vi "App - analyze RUS V6.vi"() -> ()   [LabVIEW 2018] (continued)
5_Cooling_2nd_try/September_2014/091614/102.64400K_500_2500_2.10000V_0.00000T_Sep16-2014__21-41-37_001_091614.bin", "last mod"=timestamp(3493762897 s since 1904-01-01), "file name str"="D:\\Data\\Ultrasound\\LSCO\\LSCO22__130814c\\5_Cooling_2nd_try\\September_2014\\091614\\102.64400K_500_2500_2.10000V_0.00000T_Sep16-2014__21-41-37_001_091614.bin", "mod time(min)"=58229381.61666667, "file format"=enum."binary", "power(V)"=2.1, "Magn Field(T) "=0.0}, {"temperature"=102.47, "temperature str"="102.47000", "file path"=path "D:/Data/Ultrasound/LSCO/LSCO22__130814c/5_Cooling_2nd_try/September_2014/091614/102.47000K_500_2500_2.10000V_0.00000T_Sep16-2014__21-42-56_001_091614.bin", "last mod"=timestamp(3493762976 s since 1904-01-01), "file name str"="D:\\Data\\Ultrasound\\LSCO\\LSCO22__130814c\\5_Cooling_2nd_try\\September_2014\\091614\\102.47000K_500_2500_2.10000V_0.00000T_Sep16-2014__21-42-56_001_091614.bin", "mod time(min)"=58229382.93333333, "file format"=enum."binary", "power(V)"=2.1, "Magn Field(T) "=0.0}, {"temperature"=102.285, "temperature str"="102.28500", "file path"=path "D:/Data/Ultrasound/LSCO/LSCO22__130814c/5_Cooling_2nd_try/September_2014/091614/102.28500K_500_2500_2.10000V_0.00000T_Sep16-2014__21-44-15_001_091614.bin", "last mod"=timestamp(3493763055 s since 1904-01-01), "file name str"="D:\\Data\\Ultrasound\\LSCO\\LSCO22__130814c\\5_Cooling_2nd_try\\September_2014\\091614\\102.28500K_500_2500_2.10000V_0.00000T_Sep16-2014__21-44-15_001_091614.bin", "mod time(min)"=58229384.25, "file format"=enum."binary", "power(V)"=2.1, "Magn Field(T) "=0.0}, {"temperature"=102.107, "temperature str"="102.10700", "file path"=path "D:/Data/Ultrasound/LSCO/LSCO22__130814c/5_Cooling_2nd_try/September_2014/091614/102.10700K_500_2500_2.10000V_0.00000T_Sep16-2014__21-45-35_001_091614.bin", "last mod"=timestamp(3493763135 s since 1904-01-01), "file name str"="D:\\Data\\Ultrasound\\LSCO\\LSCO22__130814c\\5_Cooling_2nd_try\\September_2014\\091614\\102.10700K_500_2500_2.10000V_0.00000T_Sep16-2014__21-45-35_001_091614.bin", "mod time(min)"=58229385.583333336, "file format"=enum."binary", "power(V)"=2.1, "Magn Field(T) "=0.0}, {"temperature"=101.933, "temperature str"="101.93300", "file path"=path "D:/Data/Ultrasound/LSCO/LSCO22__130814c/5_Cooling_2nd_try/September_2014/091614/101.93300K_500_2500_2.10000V_0.00000T_Sep16-2014__21-46-54_001_091614.bin", "last mod"=timestamp(3493763214 s since 1904-01-01), "file name str"="D:\\Data\\Ultrasound\\LSCO\\LSCO22__130814c\\5_Cooling_2nd_try\\September_2014\\091614\\101.93300K_500_2500_2.10000V_0.00000T_Sep16-2014__21-46-54_001_091614.bin", "mod time(min)"=58229386.9, "file format"=enum."binary", "power(V)"=2.1, "Magn Field(T) "=0.0}, {"temperature"=101.753, "temperature str"="101.75300", "file path"=path "D:/Data/Ultrasound/LSCO/LSCO22__130814c/5_Cooling_2nd_try/September_2014/091614/101.75300K_500_2500_2.10000V_0.00000T_Sep16-2014__21-48-14_001_091614.bin", "last mod"=timestamp(3493763294 s since 1904-01-01), "file name str"="D:\\Data\\Ultrasound\\LSCO\\LSCO22__130814c\\5_Cooling_2nd_try\\September_2014\\091614\\101.75300K_500_2500_2.10000V_0.00000T_Sep16-2014__21-48-14_001_091614.bin", "mod time(min)"=58229388.233333334, "file format"=enum."binary", "power(V)"=2.1, "Magn Field(T) "=0.0}, {"temperature"=101.581, "temperature str"="101.58100", "file path"=path "D:/Data/Ultrasound/LSCO/LSCO22__130814c/5_Cooling_2nd_try/September_2014/091614/101.58100K_500_2500_2.10000V_0.00000T_Sep16-2014__21-49-33_001_091614.bin", "last mod"=timestamp(3493763373 s since 1904-01-01), "file name str"="D:\\Data\\Ultrasound\\LSCO\\LSCO22__130814c\\5_Cooling_2nd_try\\September_2014\\091614\\101.58100K_500_2500_2.10000V_0.00000T_Sep16-2014__21-49-33_001_091614.bin", "mod time(min)"=58229389.55, "file format"=enum."binary", "power(V)"=2.1, "Magn Field(T) "=0.0}, {"temperature"=101.405, "temperature str"="101.40500", "file path"=path "D:/Data/Ultrasound/LSCO/LSCO22__130814c/5_Cooling_2nd_try/September_2014/091614/101.40500K_500_2500_2.10000V_0.00000T_Sep16-2014__21-50-52_001_091614.bin", "last mod"=timestamp(3493763452 s since 1904-01-01), "file name str"="D:\\Data\\Ultrasound\\LSCO\\LSCO22__130814c\\5_Cooling_2nd_try\\September_2014\\091614\\101.40500K_500_2500_2.10000V_0.00000T_Sep16-2014__21-50-52_001_091614.bin", "mod time(min)"=58229390.86666667, "file format"=enum."binary", "power(V)"=2.1, "Magn Field(T) "=0.0}, {"temperature"=101.228, "temperature str"="101.22800", "file path"=path "D:/Data/Ultrasound/LSCO/LSCO22__130814c/5_Cooling_2nd_try/September_2014/091614/101.22800K_500_2500_2.10000V_0.00000T_Sep16-2014__21-52-12_001_091614.bin", "last mod"=timestamp(3493763532 s since 1904-01-01), "file name str"="D:\\Data\\Ultrasound\\LSCO\\LSCO22__130814c\\5_Cooling_2nd_try\\September_2014\\091614\\101.22800K_500_2500_2.10000V_0.00000T_Sep16-2014__21-52-12_001_091614.bin", "mod time(min)"=58229392.2, "file format"=enum."binary", "power(V)"=2.1, "Magn Field(T) "=0.0}, {"temperature"=101.06, "temperature str"="101.06000", "file path"=path "D:/Data/Ultrasound/LSCO/LSCO22__130814c/5_Cooling_2nd_try/September_2014/091614/101.06000K_500_2500_2.10000V_0.00000T_Sep16-2014__21-53-31_001_091614.bin", "last mod"=timestamp(3493763611 s since 1904-01-01), "file name str"="D:\\Data\\Ultrasound\\LSCO\\LSCO22__130814c\\5_Cooling_2nd_try\\September_2014\\091614\\101.06000K_500_2500_2.10000V_0.00000T_Sep16-2014__21-53-31_001_091614.bin", "mod time(min)"=58229393.516666666, "file format"=enum."binary", "power(V)"=2.1, "Magn Field(T) "=0.0}, {"temperature"=100.883, "temperature str"="100.88300", "file path"=path "D:/Data/Ultrasound/LSCO/LSCO22__130814c/5_Cooling_2nd_try/September_2014/091614/100.88300K_500_2500_2.10000V_0.00000T_Sep16-2014__21-54-50_001_091614.bin", "last mod"=timestamp(3493763690 s since 1904-01-01), "file name str"="D:\\Data\\Ultrasound\\LSCO\\LSCO22__130814c\\5_Cooling_2nd_try\\September_2014\\091614\\100.88300K_500_2500_2.10000V_0.00000T_Sep16-2014__21-54-50_001_091614.bin", "mod time(min)"=58229394.833333336, "file format"=enum."binary", "power(V)"=2.1, "Magn Field(T) "=0.0}, {"temperature"=100.708, "temperature str"="100.70800", "file path"=path "D:/Data/Ultrasound/LSCO/LSCO22__130814c/5_Cooling_2nd_try/September_2014/091614/100.70800K_500_2500_2.10000V_0.00000T_Sep16-2014__21-56-10_001_091614.bin", "last mod"=timestamp(3493763770 s since 1904-01-01), "file name str"="D:\\Data\\Ultrasound\\LSCO\\LSCO22__130814c\\5_Cooling_2nd_try\\September_2014\\091614\\100.70800K_500_2500_2.10000V_0.00000T_Sep16-2014__21-56-10_001_091614.bin", "mod time(min)"=58229396.166666664, "file format"=enum."binary", "power(V)"=2.1, "Magn Field(T) "=0.0}, {"temperature"=100.542, "temperature str"="100.54200", "file path"=path "D:/Data/Ultrasound/LSCO/LSCO22__130814c/5_Cooling_2nd_try/September_2014/091614/100.54200K_500_2500_2.10000V_0.00000T_Sep16-2014__21-57-29_001_091614.bin", "last mod"=timestamp(3493763849 s since 1904-01-01), "file name str"="D:\\Data\\Ultrasound\\LSCO\\LSCO22__130814c\\5_Cooling_2nd_try\\September_2014\\091614\\100.54200K_500_2500_2.10000V_0.00000T_Sep16-2014__21-57-29_001_091614.bin", "mod time(min)"=58229397.483333334, "file format"=enum."binary", "power(V)"=2.1, "Magn Field(T) "=0.0}, {"temperature"=100.369, "temperature str"="100.36900", "file path"=path "D:/Data/Ultrasound/LSCO/LSCO22__130814c/5_Cooling_2nd_try/September_2014/091614/100.36900K_500_2500_2.10000V_0.00000T_Sep16-2014__21-58-49_001_091614.bin", "last mod"=timestamp(3493763929 s since 1904-01-01), "file name str"="D:\\Data\\Ultrasound\\LSCO\\LSCO22__130814c\\5_Cooling_2nd_try\\September_2014\\091614\\100.36900K_500_2500_2.10000V_0.00000T_Sep16-2014__21-58-49_001_091614.bin", "mod time(min)"=58229398.81666667, "file format"=enum."binary", "power(V)"=2.1, "Magn Field(T) "=0.0}, {"temperature"=100.203, "temperature str"="100.20300", "file path"=path "D:/Data/Ultrasound/LSCO/LSCO22__130814c/5_Cooling_2nd_try/September_2014/091614/100.20300K_500_2500_2.10000V_0.00000T_Sep16-2014__22-00-08_001_091614.bin", "last mod"=timestamp(3493764008 s since 1904-01-01), "file name str"="D:\\Data\\Ultrasound\\LSCO\\LSCO22__130814c\\5_Cooling_2nd_try\\September_2014\\091614\\100.20300K_500_2500_2.10000V_0.00000T_Sep16-2014__22-00-08_001_091614.bin", "mod time(min)"=58229400.13333333, "file format"=enum."binary", "power(V)"=2.1, "Magn Field(T) "=0.0}, {"temperature"=100.032, "temperature str"="100.03200", "file path"=path "D:/Data/Ultrasound/LSCO/LSCO22__130814c/5_Cooling_2nd_try/September_2014/091614/100.03200K_500_2500_2.10000V_0.00000T_Sep16-2014__22-01-27_001_091614.bin", "last mod"=timestamp(3493764087 s since 1904-01-01), "file name str"="D:\\Data\\Ultrasound\\LSCO\\LSCO22__130814c\\5_Cooling_2nd_try\\September_2014\\091614\\100.03200K_500_2500_2.10000V_0.00000T_Sep16-2014__22-01-27_001_091614.bin", "mod time(min)"=58229401.45, "file format"=enum."binary", "power(V)"=2.1, "Magn Field(T) "=0.0}, {"temperature"=99.859, "temperature str"="99.85900", "file path"=path "D:/Data/Ultrasound/LSCO/LSCO22__130814c/5_Cooling_2nd_try/September_2014/091614/99.85900K_500_2500_2.10000V_0.00000T_Sep16-2014__22-02-47_001_091614.bin", "last mod"=timestamp(3493764167 s since 1904-01-01), "file name str"="D:\\Data\\Ultrasound\\LSCO\\LSCO22__130814c\\5_Cooling_2nd_try\\September_2014\\091614\\99.85900K_500_2500_2.10000V_0.00000T_Sep16-2014__22-02-47_001_091614.bin", "mod time(min)"=58229402.78333333, "file format"=enum."binary", "power(V)"=2.1, "Magn Field(T) "=0.0}, {"temperature"=99.697, "temperature str"="99.69700", "file path"=path "D:/Data/Ultrasound/LSCO/LSCO22__130814c/5_Cooling_2nd_try/September_2014/091614/99.69700K_500_2500_2.10000V_0.00000T_Sep16-2014__22-04-06_001_091614.bin", "last mod"=timestamp(3493764246 s since 1904-01-01), "file name str"="D:\\Data\\Ultrasound\\LSCO\\LSCO22__130814c\\5_Cooling_2nd_try\\September_2014\\091614\\99.69700K_500_2500_2.10000V_0.00000T_Sep16-2014__22-04-06_001_091614.bin", "mod time(min)"=58229404.1, "file format"=enum."binary", "power(V)"=2.1, "Magn Field(T) "=0.0}, {"temperature"=99.53, "temperature str"="99.53000", "file path"=path "D:/Data/Ultrasound/LSCO/LSCO22__130814c/5_Cooling_2nd_try/September_2014/091614/99.53000K_500_2500_2.10000V_0.00000T_Sep16-2014__22-05-25_001_091614.bin", "last mod"=timestamp(3493764325 s since 1904-01-01), "file name str"="D:\\Data\\Ultrasound\\LSCO\\LSCO22__130814c\\5_Cooling_2nd_try\\September_2014\\091614\\99.53000K_500_2500_2.10000V_0.00000T_Sep16-2014__22-05-25_001_091614.bin", "mod time(min)"=58229405.416666664, "file format"=enum."binary", "power(V)"=2.1, "Magn Field(T) "=0.0}, {"temperature"=99.368, "temperature str"="99.36800", "file path"=path "D:/Data/Ultrasound/LSCO/LSCO22__130814c/5_Cooling_2nd_try/September_2014/091614/99.36800K_500_2500_2.10000V_0.00000T_Sep16-2014__22-06-45_001_091614.bin", "last mod"=timestamp(3493764405 s since 1904-01-01), "file name str"="D:\\Data\\Ultrasound\\LSCO\\LSCO22__130814c\\5_Cooling_2nd_try\\September_2014\\091614\\99.36800K_500_2500_2.10000V_0.00000T_Sep16-2014__22-06-45_001_091614.bin", "mod time(min)"=58229406.75, "file format"=enum."binary", "power(V)"=2.1, "Magn Field(T) "=0.0}, {"temperature"=99.199, "temperature str"="99.19900", "file path"=path "D:/Data/Ultrasound/LSCO/LSCO22__130814c/5_Cooling_2nd_try/September_2014/091614/99.19900K_500_2500_2.10000V_0.00000T_Sep16-2014__22-08-04_001_091614.bin", "last mod"=timestamp(3493764484 s since 1904-01-01), "file name str"="D:\\Data\\Ultrasound\\LSCO\\LSCO22__130814c\\5_Cooling_2nd_try\\September_2014\\091614\\99.19900K_500_2500_2.10000V_0.00000T_Sep16-2014__22-08-04_001_091614.bin", "mod time(min)"=58229408.06666667, "file format"=enum."binary", "power(V)"=2.1, "Magn Field(T) "=0.0}, {"temperature"=99.032, "temperature str"="99.03200", "file path"=path "D:/Data/Ultrasound/LSCO/LSCO22__130814c/5_Cooling_2nd_try/September_2014/091614/99.03200K_500_2500_2.10000V_0.00000T_Sep16-2014__22-09-24_001_091614.bin", "last mod"=timestamp(3493764564 s since 1904-01-01), "file name str"="D:\\Data\\Ultrasound\\LSCO\\LSCO22__130814c\\5_Cooling_2nd_try\\September_2014\\091614\\99.03200K_500_2500_2.10000V_0.00000T_Sep16-2014__22-09-24_001_091614.bin", "mod time(min)"=58229409.4, "file format"=enum."binary", "power(V)"=2.1, "Magn Field(T) "=0.0}, {"temperature"=98.874, "temperature str"="98.87400", "file path"=path "D:/Data/Ultrasound/LSCO/LSCO22__130814c/5_Cooling_2nd_try/September_2014/091614/98.87400K_500_2500_2.10000V_0.00000T_Sep16-2014__22-10-43_001_091614.bin", "last mod"=timestamp(3493764643 s since 1904-01-01), "file name str"="D:\\Data\\Ultrasound\\LSCO\\LSCO22__130814c\\5_Cooling_2nd_try\\September_2014\\091614\\98.87400K_500_2500_2.10000V_0.00000T_Sep16-2014__22-10-43_001_091614.bin", "mod time(min)"=58229410.71666667, "file format"=enum."binary", "power(V)"=2.1, "Magn Field(T) "=0.0}, {"temperature"=98.708, "temperature str"="98.70800", "file path"=path "D:/Data/Ultrasound/LSCO/LSCO22__130814c/5_Cooling_2nd_try/September_2014/091614/98.70800K_500_2500_2.10000V_0.00000T_Sep16-2014__22-12-02_001_091614.bin", "last mod"=timestamp(3493764722 s since 1904-01-01), "file name str"="D:\\Data\\Ultrasound\\LSCO\\LSCO22__130814c\\5_Cooling_2nd_try\\September_2014\\091614\\98.70800K_500_2500_2.10000V_0.00000T_Sep16-2014__22-12-02_001_091614.bin", "mod time(min)"=58229412.03333333, "file format"=enum."binary", "power(V)"=2.1, "Magn Field(T) "=0.0}, {"temperature"=98.551, "temperature str"="98.55100", "file path"=path "D:/Data/Ultrasound/LSCO/LSCO22__130814c/5_Cooling_2nd_try/September_2014/091614/98.55100K_500_2500_2.10000V_0.00000T_Sep16-2014__22-13-22_001_091614.bin", "last mod"=timestamp(3493764802 s since 1904-01-01), "file name str"="D:\\Data\\Ultrasound\\LSCO\\LSCO22__130814c\\5_Cooling_2nd_try\\September_2014\\091614\\98.55100K_500_2500_2.10000V_0.00000T_Sep16-2014__22-13-22_001_091614.bin", "mod time(min)"=58229413.36666667, "file format"=enum."binary", "power(V)"=2.1, "Magn Field(T) "=0.0}, {"temperature"=98.387, "temperature str"="98.38700", "file path"=path "D:/Data/Ultrasound/LSCO/LSCO22__130814c/5_Cooling_2nd_try/September_2014/091614/98.38700K_500_2500_2.10000V_0.00000T_Sep16-2014__22-14-41_001_091614.bin", "last mod"=timestamp(3493764881 s since 1904-01-01), "file name str"="D:\\Data\\Ultrasound\\LSCO\\LSCO22__130814c\\5_Cooling_2nd_try\\September_2014\\091614\\98.38700K_500_2500_2.10000V_0.00000T_Sep16-2014__22-14-41_001_091614.bin", "mod time(min)"=58229414.68333333, "file format"=enum."binary", "power(V)"=2.1, "Magn Field(T) "=0.0}, {"temperature"=98.223, "temperature str"="98.22300", "file path"=path "D:/Data/Ultrasound/LSCO/LSCO22__130814c/5_Cooling_2nd_try/September_2014/091614/98.22300K_500_2500_2.10000V_0.00000T_Sep16-2014__22-16-00_001_091614.bin", "last mod"=timestamp(3493764960 s since 1904-01-01), "file name str"="D:\\Data\\Ultrasound\\LSCO\\LSCO22__130814c\\5_Cooling_2nd_try\\September_2014\\091614\\98.22300K_500_2500_2.10000V_0.00000T_Sep16-2014__22-16-00_001_091614.bin", "mod time(min)"=58229416.0, "file format"=enum."binary", "power(V)"=2.1, "Magn Field(T) "=0.0}, {"temperature"=98.065, "temperature str"="98.06500", "file path"=path "D:/Data/Ultrasound/LSCO/LSCO22__130814c/5_Cooling_2nd_try/September_2014/091614/98.06500K_500_2500_2.10000V_0.00000T_Sep16-2014__22-17-20_001_091614.bin", "last mod"=timestamp(3493765040 s since 1904-01-01), "file name str"="D:\\Data\\Ultrasound\\LSCO\\LSCO22__130814c\\5_Cooling_2nd_try\\September_2014\\091614\\98.06500K_500_2500_2.10000V_0.00000T_Sep16-2014__22-17-20_001_091614.bin", "mod time(min)"=58229417.333333336, "file format"=enum."binary", "power(V)"=2.1, "Magn Field(T) "=0.0}, {"temperature"=97.905, "temperature str"="97.90500", "file path"=path "D:/Data/Ultrasound/LSCO/LSCO22__130814c/5_Cooling_2nd_try/September_2014/091614/97.90500K_500_2500_2.10000V_0.00000T_Sep16-2014__22-18-39_001_091614.bin", "last mod"=timestamp(3493765119 s since 1904-01-01), "file name str"="D:\\Data\\Ultrasound\\LSCO\\LSCO22__130814c\\5_Cooling_2nd_try\\September_2014\\091614\\97.90500K_500_2500_2.10000V_0.00000T_Sep16-2014__22-18-39_001_091614.bin", "mod time(min)"=58229418.65, "file format"=enum."binary", "power(V)"=2.1, "Magn Field(T) "=0.0}, {"temperature"=97.749, "temperature str"="97.74900", "file path"=path "D:/Data/Ultrasound/LSCO/LSCO22__130814c/5_Cooling_2nd_try/September_2014/091614/97.74900K_500_2500_2.10000V_0.00000T_Sep16-2014__22-19-59_001_091614.bin", "last mod"=timestamp(3493765199 s since 1904-01-01), "file name str"="D:\\Data\\Ultrasound\\LSCO\\LSCO22__130814c\\5_Cooling_2nd_try\\September_2014\\091614\\97.74900K_500_2500_2.10000V_0.00000T_Sep16-2014__22-19-59_001_091614.bin", "mod time(min)"=58229419.983333334, "file format"=enum."binary", "power(V)"=2.1, "Magn Field(T) "=0.0}, {"temperature"=97.59, "temperature str"="97.59000", "file path"=path "D:/Data/Ultrasound/LSCO/LSCO22__130814c/5_Cooling_2nd_try/September_2014/091614/97.59000K_500_2500_2.10000V_0.00000T_Sep16-2014__22-21-18_001_091614.bin", "last mod"=timestamp(3493765278 s since 1904-01-01), "file name str"="D:\\Data\\Ultrasound\\LSCO\\LSCO22__130814c\\5_Cooling_2nd_try\\September_2014\\091614\\97.59000K_500_2500_2.10000V_0.00000T_Sep16-2014__22-21-18_001_091614.bin", "mod time(min)"=58229421.3, "file format"=enum."binary", "power(V)"=2.1, "Magn Field(T) "=0.0}, {"temperature"=97.43, "temperature str"="97.43000", "file path"=path "D:/Data/Ultrasound/LSCO/LSCO22__130814c/5_Cooling_2nd_try/September_2014/091614/97.43000K_500_2500_2.10000V_0.00000T_Sep16-2014__22-22-37_001_091614.bin", "last mod"=timestamp(3493765357 s since 1904-01-01), "file name str"="D:\\Data\\Ultrasound\\LSCO\\LSCO22__130814c\\5_Cooling_2nd_try\\September_2014\\091614\\97.43000K_500_2500_2.10000V_0.00000T_Sep16-2014__22-22-37_001_091614.bin", "mod time(min)"=58229422.61666667, "file format"=enum."binary", "power(V)"=2.1, "Magn Field(T) "=0.0}, {"temperature"=97.276, "temperature str"="97.27600", "file path"=path "D:/Data/Ultrasound/LSCO/LSCO22__130814c/5_Cooling_2nd_try/September_2014/091614/97.27600K_500_2500_2.10000V_0.00000T_Sep16-2014__22-23-57_001_091614.bin", "last mod"=timestamp(3493765437 s since 1904-01-01), "file name str"="D:\\Data\\Ultrasound\\LSCO\\LSCO22__130814c\\5_Cooling_2nd_try\\September_2014\\091614\\97.27600K_500_2500_2.10000V_0.00000T_Sep16-2014__22-23-57_001_091614.bin", "mod time(min)"=58229423.95, "file format"=enum."binary", "power(V)"=2.1, "Magn Field(T) "=0.0}, {"temperature"=97.118, "temperature str"="97.11800", "file path"=path "D:/Data/Ultrasound/LSCO/LSCO22__130814c/5_Cooling_2nd_try/September_2014/091614/97.11800K_500_2500_2.10000V_0.00000T_Sep16-2014__22-25-16_001_091614.bin", "last mod"=timestamp(3493765516 s since 1904-01-01), "file name str"="D:\\Data\\Ultrasound\\LSCO\\LSCO22__130814c\\5_Cooling_2nd_try\\September_2014\\091614\\97.11800K_500_2500_2.10000V_0.00000T_Sep16-2014__22-25-16_001_091614.bin", "mod time(min)"=58229425.266666666, "file format"=enum."binary", "power(V)"=2.1, "Magn Field(T) "=0.0}, {"temperature"=96.968, "temperature str"="96.96800", "file path"=path "D:/Data/Ultrasound/LSCO/LSCO22__130814c/5_Cooling_2nd_try/September_2014/091614/96.96800K_500_2500_2.10000V_0.00000T_Sep16-2014__22-26-35_001_091614.bin", "last mod"=timestamp(3493765595 s since 1904-01-01), "file name str"="D:\\Data\\Ultrasound\\LSCO\\LSCO22__130814c\\5_Cooling_2nd_try\\September_2014\\091614\\96.96800K_500_2500_2.10000V_0.00000T_Sep16-2014__22-26-35_001_091614.bin", "mod time(min)"=58229426.583333336, "file format"=enum."binary", "power(V)"=2.1, "Magn Field(T) "=0.0}, {"temperature"=96.812, "temperature str"="96.81200", "file path"=path "D:/Data/Ultrasound/LSCO/LSCO22__130814c/5_Cooling_2nd_try/September_2014/091614/96.81200K_500_2500_2.10000V_0.00000T_Sep16-2014__22-27-55_001_091614.bin", "last mod"=timestamp(3493765675 s since 1904-01-01), "file name str"="D:\\Data\\Ultrasound\\LSCO\\LSCO22__130814c\\5_Cooling_2nd_try\\September_2014\\091614\\96.81200K_500_2500_2.10000V_0.00000T_Sep16-2014__22-27-55_001_091614.bin", "mod time(min)"=58229427.916666664, "file format"=enum."binary", "power(V)"=2.1, "Magn Field(T) "=0.0}, {"temperature"=96.655, "temperature str"="96.65500", "file path"=path "D:/Data/Ultrasound/LSCO/LSCO22__130814c/5_Cooling_2nd_try/September_2014/091614/96.65500K_500_2500_2.10000V_0.00000T_Sep16-2014__22-29-14_001_091614.bin", "last mod"=timestamp(3493765754 s since 1904-01-01), "file name str"="D:\\Data\\Ultrasound\\LSCO\\LSCO22__130814c\\5_Cooling_2nd_try\\September_2014\\091614\\96.65500K_500_2500_2.10000V_0.00000T_Sep16-2014__22-29-14_001_091614.bin", "mod time(min)"=58229429.233333334, "file format"=enum."binary", "power(V)"=2.1, "Magn Field(T) "=0.0}, {"temperature"=96.507, "temperature str"="96.50700", "file path"=path "D:/Data/Ultrasound/LSCO/LSCO22__130814c/5_Cooling_2nd_try/September_2014/091614/96.50700K_500_2500_2.10000V_0.00000T_Sep16-2014__22-30-34_001_091614.bin", "last mod"=timestamp(3493765834 s since 1904-01-01), "file name str"="D:\\Data\\Ultrasound\\LSCO\\LSCO22__130814c\\5_Cooling_2nd_try\\September_2014\\091614\\96.50700K_500_2500_2.10000V_0.00000T_Sep16-2014__22-30-34_001_091614.bin", "mod time(min)"=58229430.56666667, "file format"=enum."binary", "power(V)"=2.1, "Magn Field(T) "=0.0}, {"temperature"=96.351, "temperature str"="96.35100", "file path"=path "D:/Data/Ultrasound/LSCO/LSCO22__130814c/5_Cooling_2nd_try/September_2014/091614/96.35100K_500_2500_2.10000V_0.00000T_Sep16-2014__22-31-53_001_091614.bin", "last mod"=timestamp(3493765913 s since 1904-01-01), "file name str"="D:\\Data\\Ultrasound\\LSCO\\LSCO22__130814c\\5_Cooling_2nd_try\\September_2014\\091614\\96.35100K_500_2500_2.10000V_0.00000T_Sep16-2014__22-31-53_001_091614.bin", "mod time(min)"=58229431.88333333, "file format"=enum."binary", "power(V)"=2.1, "Magn Field(T) "=0.0}, {"temperature"=96.204, "temperature str"="96.20400", "file path"=path "D:/Data/Ultrasound/LSCO/LSCO22__130814c/5_Cooling_2nd_try/September_2014/091614/96.20400K_500_2500_2.10000V_0.00000T_Sep16-2014__22-33-12_001_091614.bin", "last mod"=timestamp(3493765992 s since 1904-01-01), "file name str"="D:\\Data\\Ultrasound\\LSCO\\LSCO22__130814c\\5_Cooling_2nd_try\\September_2014\\091614\\96.20400K_500_2500_2.10000V_0.00000T_Sep16-2014__22-33-12_001_091614.bin", "mod time(min)"=58229433.2, "file format"=enum."binary", "power(V)"=2.1, "Magn Field(T) "=0.0}, {"temperature"=96.051, "temperature str"="96.05100", "file path"=path "D:/Data/Ultrasound/LSCO/LSCO22__130814c/5_Cooling_2nd_try/September_2014/091614/96.05100K_500_2500_2.10000V_0.00000T_Sep16-2014__22-34-32_001_091614.bin", "last mod"=timestamp(3493766072 s since 1904-01-01), "file name str"="D:\\Data\\Ultrasound\\LSCO\\LSCO22__130814c\\5_Cooling_2nd_try\\September_2014\\091614\\96.05100K_500_2500_2.10000V_0.00000T_Sep16-2014__22-34-32_001_091614.bin", "mod time(min)"=58229434.53333333, "file format"=enum."binary", "power(V)"=2.1, "Magn Field(T) "=0.0}, {"temperature"=95.897, "temperature str"="95.89700", "file path"=path "D:/Data/Ultrasound/LSCO/LSCO22__130814c/5_Cooling_2nd_try/September_2014/091614/95.89700K_500_2500_2.10000V_0.00000T_Sep16-2014__22-35-51_001_091614.bin", "last mod"=timestamp(3493766151 s since 1904-01-01), "file name str"="D:\\Data\\Ultrasound\\LSCO\\LSCO22__130814c\\5_Cooling_2nd_try\\September_2014\\091614\\95.89700K_500_2500_2.10000V_0.00000T_Sep16-2014__22-35-51_001_091614.bin", "mod time(min)"=58229435.85, "file format"=enum."binary", "power(V)"=2.1, "Magn Field(T) "=0.0}, {"temperature"=95.75, "temperature str"="95.75000", "file path"=path "D:/Data/Ultrasound/LSCO/LSCO22__130814c/5_Cooling_2nd_try/September_2014/091614/95.75000K_500_2500_2.10000V_0.00000T_Sep16-2014__22-37-10_001_091614.bin", "last mod"=timestamp(3493766230 s since 1904-01-01), "file name str"="D:\\Data\\Ultrasound\\LSCO\\LSCO22__130814c\\5_Cooling_2nd_try\\September_2014\\091614\\95.75000K_500_2500_2.10000V_0.00000T_Sep16-2014__22-37-10_001_091614.bin", "mod time(min)"=58229437.166666664, "file format"=enum."binary", "power(V)"=2.1, "Magn Field(T) "=0.0}, {"temperature"=95.599, "temperature str"="95.59900", "file path"=path "D:/Data/Ultrasound/LSCO/LSCO22__130814c/5_Cooling_2nd_try/September_2014/091614/95.59900K_500_2500_2.10000V_0.00000T_Sep16-2014__22-38-30_001_091614.bin", "last mod"=timestamp(3493766310 s since 1904-01-01), "file name str"="D:\\Data\\Ultrasound\\LSCO\\LSCO22__130814c\\5_Cooling_2nd_try\\September_2014\\091614\\95.59900K_500_2500_2.10000V_0.00000T_Sep16-2014__22-38-30_001_091614.bin", "mod time(min)"=58229438.5, "file format"=enum."binary", "power(V)"=2.1, "Magn Field(T) "=0.0}, {"temperature"=95.455, "temperature str"="95.45500", "file path"=path "D:/Data/Ultrasound/LSCO/LSCO22__130814c/5_Cooling_2nd_try/September_2014/091614/95.45500K_500_2500_2.10000V_0.00000T_Sep16-2014__22-39-49_001_091614.bin", "last mod"=timestamp(3493766389 s since 1904-01-01), "file name str"="D:\\Data\\Ultrasound\\LSCO\\LSCO22__130814c\\5_Cooling_2nd_try\\September_2014\\091614\\95.45500K_500_2500_2.10000V_0.00000T_Sep16-2014__22-39-49_001_091614.bin", "mod time(min)"=58229439.81666667, "file format"=enum."binary", "power(V)"=2.1, "Magn Field(T) "=0.0}, {"temperature"=95.306, "temperature str"="95.30600", "file path"=path "D:/Data/Ultrasound/LSCO/LSCO22__130814c/5_Cooling_2nd_try/September_2014/091614/95.30600K_500_2500_2.10000V_0.00000T_Sep16-2014__22-41-08_001_091614.bin", "last mod"=timestamp(3493766468 s since 1904-01-01), "file name str"="D:\\Data\\Ultrasound\\LSCO\\LSCO22__130814c\\5_Cooling_2nd_try\\September_2014\\091614\\95.30600K_500_2500_2.10000V_0.00000T_Sep16-2014__22-41-08_001_091614.bin", "mod time(min)"=58229441.13333333, "file format"=enum."binary", "power(V)"=2.1, "Magn Field(T) "=0.0}, {"temperature"=95.156, "temperature str"="95.15600", "file path"=path "D:/Data/Ultrasound/LSCO/LSCO22__130814c/5_Cooling_2nd_try/September_2014/091614/95.15600K_500_2500_2.10000V_0.00000T_Sep16-2014__22-42-28_001_091614.bin", "last mod"=timestamp(3493766548 s since 1904-01-01), "file name str"="D:\\Data\\Ultrasound\\LSCO\\LSCO22__130814c\\5_Cooling_2nd_try\\September_2014\\091614\\95.15600K_500_2500_2.10000V_0.00000T_Sep16-2014__22-42-28_001_091614.bin", "mod time(min)"=58229442.46666667, "file format"=enum."binary", "power(V)"=2.1, "Magn Field(T) "=0.0}, {"temperature"=95.012, "temperature str"="95.01200", "file path"=path "D:/Data/Ultrasound/LSCO/LSCO22__130814c/5_Cooling_2nd_try/September_2014/091614/95.01200K_500_2500_2.10000V_0.00000T_Sep16-2014__22-43-47_001_091614.bin", "last mod"=timestamp(3493766627 s since 1904-01-01), "file name str"="D:\\Data\\Ultrasound\\LSCO\\LSCO22__130814c\\5_Cooling_2nd_try\\September_2014\\091614\\95.01200K_500_2500_2.10000V_0.00000T_Sep16-2014__22-43-47_001_091614.bin", "mod time(min)"=58229443.78333333, "file format"=enum."binary", "power(V)"=2.1, "Magn Field(T) "=0.0}, {"temperature"=94.866, "temperature str"="94.86600", "file path"=path "D:/Data/Ultrasound/LSCO/LSCO22__130814c/5_Cooling_2nd_try/September_2014/091614/94.86600K_500_2500_2.10000V_0.00000T_Sep16-2014__22-45-07_001_091614.bin", "last mod"=timestamp(3493766707 s since 1904-01-01), "file name str"="D:\\Data\\Ultrasound\\LSCO\\LSCO22__130814c\\5_Cooling_2nd_try\\September_2014\\091614\\94.86600K_500_2500_2.10000V_0.00000T_Sep16-2014__22-45-07_001_091614.bin", "mod time(min)"=58229445.11666667, "file format"=enum."binary", "power(V)"=2.1, "Magn Field(T) "=0.0}, {"temperature"=94.718, "temperature str"="94.71800", "file path"=path "D:/Data/Ultrasound/LSCO/LSCO22__130814c/5_Cooling_2nd_try/September_2014/091614/94.71800K_500_2500_2.10000V_0.00000T_Sep16-2014__22-46-26_001_091614.bin", "last mod"=timestamp(3493766786 s since 1904-01-01), "file name str"="D:\\Data\\Ultrasound\\LSCO\\LSCO22__130814c\\5_Cooling_2nd_try\\September_2014\\091614\\94.71800K_500_2500_2.10000V_0.00000T_Sep16-2014__22-46-26_001_091614.bin", "mod time(min)"=58229446.43333333, "file format"=enum."binary", "power(V)"=2.1, "Magn Field(T) "=0.0}, {"temperature"=94.578, "temperature str"="94.57800", "file path"=path "D:/Data/Ultrasound/LSCO/LSCO22__130814c/5_Cooling_2nd_try/September_2014/091614/94.57800K_500_2500_2.10000V_0.00000T_Sep16-2014__22-47-45_001_091614.bin", "last mod"=timestamp(3493766865 s since 1904-01-01), "file name str"="D:\\Data\\Ultrasound\\LSCO\\LSCO22__130814c\\5_Cooling_2nd_try\\September_2014\\091614\\94.57800K_500_2500_2.10000V_0.00000T_Sep16-2014__22-47-45_001_091614.bin", "mod time(min)"=58229447.75, "file format"=enum."binary", "power(V)"=2.1, "Magn Field(T) "=0.0}, {"temperature"=94.43, "temperature str"="94.43000", "file path"=path "D:/Data/Ultrasound/LSCO/LSCO22__130814c/5_Cooling_2nd_try/September_2014/091614/94.43000K_500_2500_2.10000V_0.00000T_Sep16-2014__22-49-05_001_091614.bin", "last mod"=timestamp(3493766945 s since 1904-01-01), "file name str"="D:\\Data\\Ultrasound\\LSCO\\LSCO22__130814c\\5_Cooling_2nd_try\\September_2014\\091614\\94.43000K_500_2500_2.10000V_0.00000T_Sep16-2014__22-49-05_001_091614.bin", "mod time(min)"=58229449.083333336, "file format"=enum."binary", "power(V)"=2.1, "Magn Field(T) "=0.0}, {"temperature"=94.292, "temperature str"="94.29200", "file path"=path "D:/Data/Ultrasound/LSCO/LSCO22__130814c/5_Cooling_2nd_try/September_2014/091614/94.29200K_500_2500_2.10000V_0.00000T_Sep16-2014__22-50-24_001_091614.bin", "last mod"=timestamp(3493767024 s since 1904-01-01), "file name str"="D:\\Data\\Ultrasound\\LSCO\\LSCO22__130814c\\5_Cooling_2nd_try\\September_2014\\091614\\94.29200K_500_2500_2.10000V_0.00000T_Sep16-2014__22-50-24_001_091614.bin", "mod time(min)"=58229450.4, "file format"=enum."binary", "power(V)"=2.1, "Magn Field(T) "=0.0}, {"temperature"=94.146, "temperature str"="94.14600", "file path"=path "D:/Data/Ultrasound/LSCO/LSCO22__130814c/5_Cooling_2nd_try/September_2014/091614/94.14600K_500_2500_2.10000V_0.00000T_Sep16-2014__22-51-43_001_091614.bin", "last mod"=timestamp(3493767103 s since 1904-01-01), "file name str"="D:\\Data\\Ultrasound\\LSCO\\LSCO22__130814c\\5_Cooling_2nd_try\\September_2014\\091614\\94.14600K_500_2500_2.10000V_0.00000T_Sep16-2014__22-51-43_001_091614.bin", "mod time(min)"=58229451.71666667, "file format"=enum."binary", "power(V)"=2.1, "Magn Field(T) "=0.0}, {"temperature"=94.003, "temperature str"="94.00300", "file path"=path "D:/Data/Ultrasound/LSCO/LSCO22__130814c/5_Cooling_2nd_try/September_2014/091614/94.00300K_500_2500_2.10000V_0.00000T_Sep16-2014__22-53-03_001_091614.bin", "last mod"=timestamp(3493767183 s since 1904-01-01), "file name str"="D:\\Data\\Ultrasound\\LSCO\\LSCO22__130814c\\5_Cooling_2nd_try\\September_2014\\091614\\94.00300K_500_2500_2.10000V_0.00000T_Sep16-2014__22-53-03_001_091614.bin", "mod time(min)"=58229453.05, "file format"=enum."binary", "power(V)"=2.1, "Magn Field(T) "=0.0}, {"temperature"=93.867, "temperature str"="93.86700", "file path"=path "D:/Data/Ultrasound/LSCO/LSCO22__130814c/5_Cooling_2nd_try/September_2014/091614/93.86700K_500_2500_2.10000V_0.00000T_Sep16-2014__22-54-22_001_091614.bin", "last mod"=timestamp(3493767262 s since 1904-01-01), "file name str"="D:\\Data\\Ultrasound\\LSCO\\LSCO22__130814c\\5_Cooling_2nd_try\\September_2014\\091614\\93.86700K_500_2500_2.10000V_0.00000T_Sep16-2014__22-54-22_001_091614.bin", "mod time(min)"=58229454.36666667, "file format"=enum."binary", "power(V)"=2.1, "Magn Field(T) "=0.0}, {"temperature"=93.722, "temperature str"="93.72200", "file path"=path "D:/Data/Ultrasound/LSCO/LSCO22__130814c/5_Cooling_2nd_try/September_2014/091614/93.72200K_500_2500_2.10000V_0.00000T_Sep16-2014__22-55-42_001_091614.bin", "last mod"=timestamp(3493767342 s since 1904-01-01), "file name str"="D:\\Data\\Ultrasound\\LSCO\\LSCO22__130814c\\5_Cooling_2nd_try\\September_2014\\091614\\93.72200K_500_2500_2.10000V_0.00000T_Sep16-2014__22-55-42_001_091614.bin", "mod time(min)"=58229455.7, "file format"=enum."binary", "power(V)"=2.1, "Magn Field(T) "=0.0}, {"temperature"=93.585, "temperature str"="93.58500", "file path"=path "D:/Data/Ultrasound/LSCO/LSCO22__130814c/5_Cooling_2nd_try/September_2014/091614/93.58500K_500_2500_2.10000V_0.00000T_Sep16-2014__22-57-01_001_091614.bin", "last mod"=timestamp(3493767421 s since 1904-01-01), "file name str"="D:\\Data\\Ultrasound\\LSCO\\LSCO22__130814c\\5_Cooling_2nd_try\\September_2014\\091614\\93.58500K_500_2500_2.10000V_0.00000T_Sep16-2014__22-57-01_001_091614.bin", "mod time(min)"=58229457.016666666, "file format"=enum."binary", "power(V)"=2.1, "Magn Field(T) "=0.0}, {"temperature"=93.444, "temperature str"="93.44400", "file path"=path "D:/Data/Ultrasound/LSCO/LSCO22__130814c/5_Cooling_2nd_try/September_2014/091614/93.44400K_500_2500_2.10000V_0.00000T_Sep16-2014__22-58-20_001_091614.bin", "last mod"=timestamp(3493767500 s since 1904-01-01), "file name str"="D:\\Data\\Ultrasound\\LSCO\\LSCO22__130814c\\5_Cooling_2nd_try\\September_2014\\091614\\93.44400K_500_2500_2.10000V_0.00000T_Sep16-2014__22-58-20_001_091614.bin", "mod time(min)"=58229458.333333336, "file format"=enum."binary", "power(V)"=2.1, "Magn Field(T) "=0.0}, {"temperature"=93.303, "temperature str"="93.30300", "file path"=path "D:/Data/Ultrasound/LSCO/LSCO22__130814c/5_Cooling_2nd_try/September_2014/091614/93.30300K_500_2500_2.10000V_0.00000T_Sep16-2014__22-59-40_001_091614.bin", "last mod"=timestamp(3493767580 s since 1904-01-01), "file name str"="D:\\Data\\Ultrasound\\LSCO\\LSCO22__130814c\\5_Cooling_2nd_try\\September_2014\\091614\\93.30300K_500_2500_2.10000V_0.00000T_Sep16-2014__22-59-40_001_091614.bin", "mod time(min)"=58229459.666666664, "file format"=enum."binary", "power(V)"=2.1, "Magn Field(T) "=0.0}, {"temperature"=93.168, "temperature str"="93.16800", "file path"=path "D:/Data/Ultrasound/LSCO/LSCO22__130814c/5_Cooling_2nd_try/September_2014/091614/93.16800K_500_2500_2.10000V_0.00000T_Sep16-2014__23-00-59_001_091614.bin", "last mod"=timestamp(3493767659 s since 1904-01-01), "file name str"="D:\\Data\\Ultrasound\\LSCO\\LSCO22__130814c\\5_Cooling_2nd_try\\September_2014\\091614\\93.16800K_500_2500_2.10000V_0.00000T_Sep16-2014__23-00-59_001_091614.bin", "mod time(min)"=58229460.983333334, "file format"=enum."binary", "power(V)"=2.1, "Magn Field(T) "=0.0}, {"temperature"=93.028, "temperature str"="93.02800", "file path"=path "D:/Data/Ultrasound/LSCO/LSCO22__130814c/5_Cooling_2nd_try/September_2014/091614/93.02800K_500_2500_2.10000V_0.00000T_Sep16-2014__23-02-18_001_091614.bin", "last mod"=timestamp(3493767738 s since 1904-01-01), "file name str"="D:\\Data\\Ultrasound\\LSCO\\LSCO22__130814c\\5_Cooling_2nd_try\\September_2014\\091614\\93.02800K_500_2500_2.10000V_0.00000T_Sep16-2014__23-02-18_001_091614.bin", "mod time(min)"=58229462.3, "file format"=enum."binary", "power(V)"=2.1, "Magn Field(T) "=0.0}, {"temperature"=92.895, "temperature str"="92.89500", "file path"=path "D:/Data/Ultrasound/LSCO/LSCO22__130814c/5_Cooling_2nd_try/September_2014/091614/92.89500K_500_2500_2.10000V_0.00000T_Sep16-2014__23-03-38_001_091614.bin", "last mod"=timestamp(3493767818 s since 1904-01-01), "file name str"="D:\\Data\\Ultrasound\\LSCO\\LSCO22__130814c\\5_Cooling_2nd_try\\September_2014\\091614\\92.89500K_500_2500_2.10000V_0.00000T_Sep16-2014__23-03-38_001_091614.bin", "mod time(min)"=58229463.63333333, "file format"=enum."binary", "power(V)"=2.1, "Magn Field(T) "=0.0}, {"temperature"=92.755, "temperature str"="92.75500", "file path"=path "D:/Data/Ultrasound/LSCO/LSCO22__130814c/5_Cooling_2nd_try/September_2014/091614/92.75500K_500_2500_2.10000V_0.00000T_Sep16-2014__23-04-57_001_091614.bin", "last mod"=timestamp(3493767897 s since 1904-01-01), "file name str"="D:\\Data\\Ultrasound\\LSCO\\LSCO22__130814c\\5_Cooling_2nd_try\\September_2014\\091614\\92.75500K_500_2500_2.10000V_0.00000T_Sep16-2014__23-04-57_001_091614.bin", "mod time(min)"=58229464.95, "file format"=enum."binary", "power(V)"=2.1, "Magn Field(T) "=0.0}, {"temperature"=92.618, "temperature str"="92.61800", "file path"=path "D:/Data/Ultrasound/LSCO/LSCO22__130814c/5_Cooling_2nd_try/September_2014/091614/92.61800K_500_2500_2.10000V_0.00000T_Sep16-2014__23-06-17_001_091614.bin", "last mod"=timestamp(3493767977 s since 1904-01-01), "file name str"="D:\\Data\\Ultrasound\\LSCO\\LSCO22__130814c\\5_Cooling_2nd_try\\September_2014\\091614\\92.61800K_500_2500_2.10000V_0.00000T_Sep16-2014__23-06-17_001_091614.bin", "mod time(min)"=58229466.28333333, "file format"=enum."binary", "power(V)"=2.1, "Magn Field(T) "=0.0}, {"temperature"=92.485, "temperature str"="92.48500", "file path"=path "D:/Data/Ultrasound/LSCO/LSCO22__130814c/5_Cooling_2nd_try/September_2014/091614/92.48500K_500_2500_2.10000V_0.00000T_Sep16-2014__23-07-36_001_091614.bin", "last mod"=timestamp(3493768056 s since 1904-01-01), "file name str"="D:\\Data\\Ultrasound\\LSCO\\LSCO22__130814c\\5_Cooling_2nd_try\\September_2014\\091614\\92.48500K_500_2500_2.10000V_0.00000T_Sep16-2014__23-07-36_001_091614.bin", "mod time(min)"=58229467.6, "file format"=enum."binary", "power(V)"=2.1, "Magn Field(T) "=0.0}, {"temperature"=92.348, "temperature str"="92.34800", "file path"=path "D:/Data/Ultrasound/LSCO/LSCO22__130814c/5_Cooling_2nd_try/September_2014/091614/92.34800K_500_2500_2.10000V_0.00000T_Sep16-2014__23-08-55_001_091614.bin", "last mod"=timestamp(3493768135 s since 1904-01-01), "file name str"="D:\\Data\\Ultrasound\\LSCO\\LSCO22__130814c\\5_Cooling_2nd_try\\September_2014\\091614\\92.34800K_500_2500_2.10000V_0.00000T_Sep16-2014__23-08-55_001_091614.bin", "mod time(min)"=58229468.916666664, "file format"=enum."binary", "power(V)"=2.1, "Magn Field(T) "=0.0}, {"temperature"=92.218, "temperature str"="92.21800", "file path"=path "D:/Data/Ultrasound/LSCO/LSCO22__130814c/5_Cooling_2nd_try/September_2014/091614/92.21800K_500_2500_2.10000V_0.00000T_Sep16-2014__23-10-15_001_091614.bin", "last mod"=timestamp(3493768215 s since 1904-01-01), "file name str"="D:\\Data\\Ultrasound\\LSCO\\LSCO22__130814c\\5_Cooling_2nd_try\\September_2014\\091614\\92.21800K_500_2500_2.10000V_0.00000T_Sep16-2014__23-10-15_001_091614.bin", "mod time(min)"=58229470.25, "file format"=enum."binary", "power(V)"=2.1, "Magn Field(T) "=0.0}, {"temperature"=92.082, "temperature str"="92.08200", "file path"=path "D:/Data/Ultrasound/LSCO/LSCO22__130814c/5_Cooling_2nd_try/September_2014/091614/92.08200K_500_2500_2.10000V_0.00000T_Sep16-2014__23-11-34_001_091614.bin", "last mod"=timestamp(3493768294 s since 1904-01-01), "file name str"="D:\\Data\\Ultrasound\\LSCO\\LSCO22__130814c\\5_Cooling_2nd_try\\September_2014\\091614\\92.08200K_500_2500_2.10000V_0.00000T_Sep16-2014__23-11-34_001_091614.bin", "mod time(min)"=58229471.56666667, "file format"=enum."binary", "power(V)"=2.1, "Magn Field(T) "=0.0}, {"temperature"=91.948, "temperature str"="91.94800", "file path"=path "D:/Data/Ultrasound/LSCO/LSCO22__130814c/5_Cooling_2nd_try/September_2014/091614/91.94800K_500_2500_2.10000V_0.00000T_Sep16-2014__23-12-53_001_091614.bin", "last mod"=timestamp(3493768373 s since 1904-01-01), "file name str"="D:\\Data\\Ultrasound\\LSCO\\LSCO22__130814c\\5_Cooling_2nd_try\\September_2014\\091614\\91.94800K_500_2500_2.10000V_0.00000T_Sep16-2014__23-12-53_001_091614.bin", "mod time(min)"=58229472.88333333, "file format"=enum."binary", "power(V)"=2.1, "Magn Field(T) "=0.0}, {"temperature"=91.818, "temperature str"="91.81800", "file path"=path "D:/Data/Ultrasound/LSCO/LSCO22__130814c/5_Cooling_2nd_try/September_2014/091614/91.81800K_500_2500_2.10000V_0.00000T_Sep16-2014__23-14-13_001_091614.bin", "last mod"=timestamp(3493768453 s since 1904-01-01), "file name str"="D:\\Data\\Ultrasound\\LSCO\\LSCO22__130814c\\5_Cooling_2nd_try\\September_2014\\091614\\91.81800K_500_2500_2.10000V_0.00000T_Sep16-2014__23-14-13_001_091614.bin", "mod time(min)"=58229474.21666667, "file format"=enum."binary", "power(V)"=2.1, "Magn Field(T) "=0.0}, {"temperature"=91.685, "temperature str"="91.68500", "file path"=path "D:/Data/Ultrasound/LSCO/LSCO22__130814c/5_Cooling_2nd_try/September_2014/091614/91.68500K_500_2500_2.10000V_0.00000T_Sep16-2014__23-15-32_001_091614.bin", "last mod"=timestamp(3493768532 s since 1904-01-01), "file name str"="D:\\Data\\Ultrasound\\LSCO\\LSCO22__130814c\\5_Cooling_2nd_t
